vi "Read VISA session.vi"(8 "error in (no error)":errorcluster, 11 "Scope VISA CFG in":refnum<class "Scope VISA CFG.lvclass">) -> (0 "error out":errorcluster, 2 "VISA session":refnum<visa-resource-name>, 3 "Scope VISA CFG out":refnum<class "Scope VISA CFG.lvclass">)   [LabVIEW 2023, in "Scope.lvlib" / "Scope VISA.lvlib" / "Scope VISA CFG.lvclass"]
uses:
  Scope VISA CFG.lvclass
  Scope VISA CFG.lvclass/Scope VISA CFG.ctl
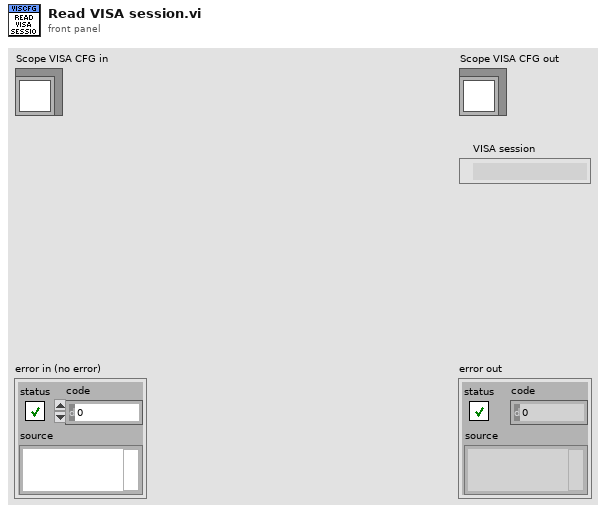
[diagram p1: front panel]
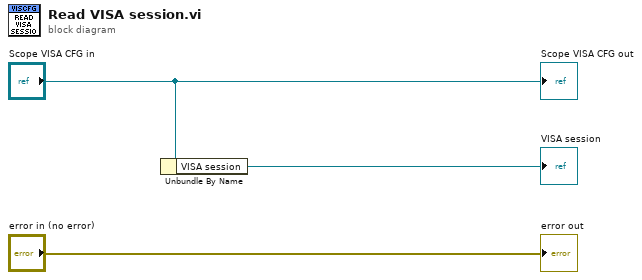
[diagram p0: block diagram]
diagram:
  n1 = Unbundle By Name("Scope VISA CFG in") -> ("VISA session"=→"VISA session":refnum<visa-resource-name>)
  "error out" <- "error in (no error)"
  "Scope VISA CFG out" <- "Scope VISA CFG in"
